vi "2 DOF Helicopter.vi"() -> ()   [LabVIEW 2021]
uses:
  <vilib>/MakerHub/LINX/Public/Sensors/Accelerometer/MPU60X0/DeviceAddresses.ctl
  <vilib>/Simulation/Scripting/Companion Diagram/SimConfigNode/SimParams.ctl
  <vilib>/Simulation/Scripting/Companion Diagram/SimConfigNode/_simSolvers.ctl
  <vilib>/Simulation/Implementation/Shared/SIMSCR Execution Mode.ctl
  <vilib>/Simulation/Param Hierarchy/Typedefs/SIMPH Param Control Actions.ctl
  <vilib>/Simulation/Implementation/Shared/SIM limit type.ctl
  <vilib>/Simulation/Implementation/Shared/NILVSim_ParamChanged.vi
  <vilib>/Simulation/Implementation/Shared/NILVSIM_BeginStep.vi
  <vilib>/Simulation/Utility/Implementation/SIM Halt.vi
  <vilib>/Simulation/SignalArithmetic/Implementation/NILVSim Gain.llb/SIM Gain (scalar).vi
  <vilib>/Simulation/ContinuousLinear/Implementation/NILVSim Derivative.llb/SIM derivative (scalar).vi
  <vilib>/Simulation/SignalDisplay/Implementation/NILVSim Time Waveform.llb/SIM Time Waveform (vector).vi
  <vilib>/Simulation/ContinuousLinear/Implementation/NILVSim Integrator new.llb/SIM Integrator distributor (scalar).vi
  <vilib>/Simulation/ContinuousLinear/Implementation/NILVSim Integrator new.llb/SIM Integrator collector (scalar).vi
  <vilib>/Simulation/Implementation/Shared/SIM Is Init or Final Stage.vi
  <vilib>/MakerHub/LINX/Public/Peripherals/Digital/Digital Write.vi
  <vilib>/MakerHub/LINX/Public/Peripherals/Digital/Digital Write 1 Chan.vi
  <vilib>/MakerHub/LINX/Public/Peripherals/PWM/PWM Set Duty Cycle.vi
  <vilib>/MakerHub/LINX/Public/Peripherals/PWM/PWM Set Duty Cycle 1 Chan.vi
  <vilib>/Simulation/Implementation/Shared/NILVSim_Manager.vi
  <vilib>/Utility/error.llb/Clear Errors.vi
  <vilib>/Simulation/Implementation/Shared/NILVSim_FinalizeModel.vi
  <vilib>/MakerHub/LINX/Public/Peripherals/Digital/Digital Write N Chans.vi
  <vilib>/MakerHub/LINX/Private/Local IO/LinxDigitalWrite.vi
  <vilib>/MakerHub/LINX/Public/Utilities/Check Channel.vi
  <vilib>/MakerHub/LINX/Public/Utilities/Open Serial.vi
  <vilib>/Simulation/Implementation/Shared/SIM Unbundle Sim Info.vi
  <vilib>/Simulation/Implementation/Shared/NILVSim_Initialize.vi
  <vilib>/MakerHub/LINX/Private/Utilties/Generate Error.vi
  <vilib>/MakerHub/LINX/Private/Device/Peripheral/Digital/Digital Write.vi
  <vilib>/MakerHub/LINX/Public/Peripherals/PWM/PWM Set Duty Cycle N Chans.vi
  <vilib>/Simulation/Utility/Implementation/NILVSim Get Time and IsAcceptedStep.vi
  <vilib>/Simulation/Implementation/Shared/SIMSH Read Queue.vi
  <vilib>/Simulation/Implementation/Shared/NILVSim_GetModelError.vi
  <vilib>/Simulation/Implementation/Shared/SIM Bundle Sim Info.vi
  <vilib>/Simulation/Scripting/Companion Diagram/SimConfigNode/SimDog.xnode
  <vilib>/Simulation/Implementation/XNodeFramework/SimXNode/SimX.xnode
  <vilib>/MakerHub/LINX/LMH-LINX.lvlib
  <vilib>/MakerHub/LINX/Public/Sensors/Accelerometer/MPU60X0/MPU60X0.lvlib
  <vilib>/Simulation/ContinuousLinear/Implementation/NILVSim Integrator new.llb/SIM Integrator (scalar).vi
  <vilib>/Simulation/Implementation/Shared/NI_SIM_Implementation.lvlib
panel:
  out "u 2":dbl
  in  "Max 2":dbl=0.9
  in  "Controller 2 ON/OFF":bool
  in  "Gain 2":dbl=15.0
  in  "Kp 2":dbl=24.0
  in  "Ki  2":dbl=1.0
  in  "Kd  2":dbl=0.1
  out "Error Out 2":errorcluster
  out "Waveform Chart":waveform(dbl)[](graph)=[{"t0"=timestamp(2.05 s since 1904-01-01), "dt"=1.0, "Y"=[0.011969439452488623]}, {"t0"=timestamp(2.05 s since 1904-01-01), "dt"=1.0, "Y"=[0.0]}]
  out "Y Axis":i16=574
  in  "Gain":dbl=1.0
  in  "Max":dbl=0.8
  in  "Controller ON/OFF":bool
  out "u":dbl
  out "Iterations":i32=1999
  in  "Iterations":i32=2000
  out "yaw":dbl=0.5188562340966918
  out "Z Axis":i16=1
  out "x/y":dbl=-89.86768864889659
  in  "Halt?":bool
  out "pitch":dbl=0.011969439452488623
  out "Gyro\n Chart 2":T1(graph)={"X Axis"=-479, "Y Axis"=574, "Z Axis"=61}
  out "Acceleration\n Chart":T1(graph)={"X Axis"=4, "Y Axis"=-2344, "Z Axis"=19140}
  out "Acceleration Data (g)":T1={"X Axis"=4, "Y Axis"=-2344, "Z Axis"=19140}
  out "Error Out":errorcluster
  in  "Serial Port":refnum<visa-resource-name>="COM7"
  in  "Kp":dbl=25.0
  in  "Ki":dbl=0.3
  in  "Kd":dbl=0.2
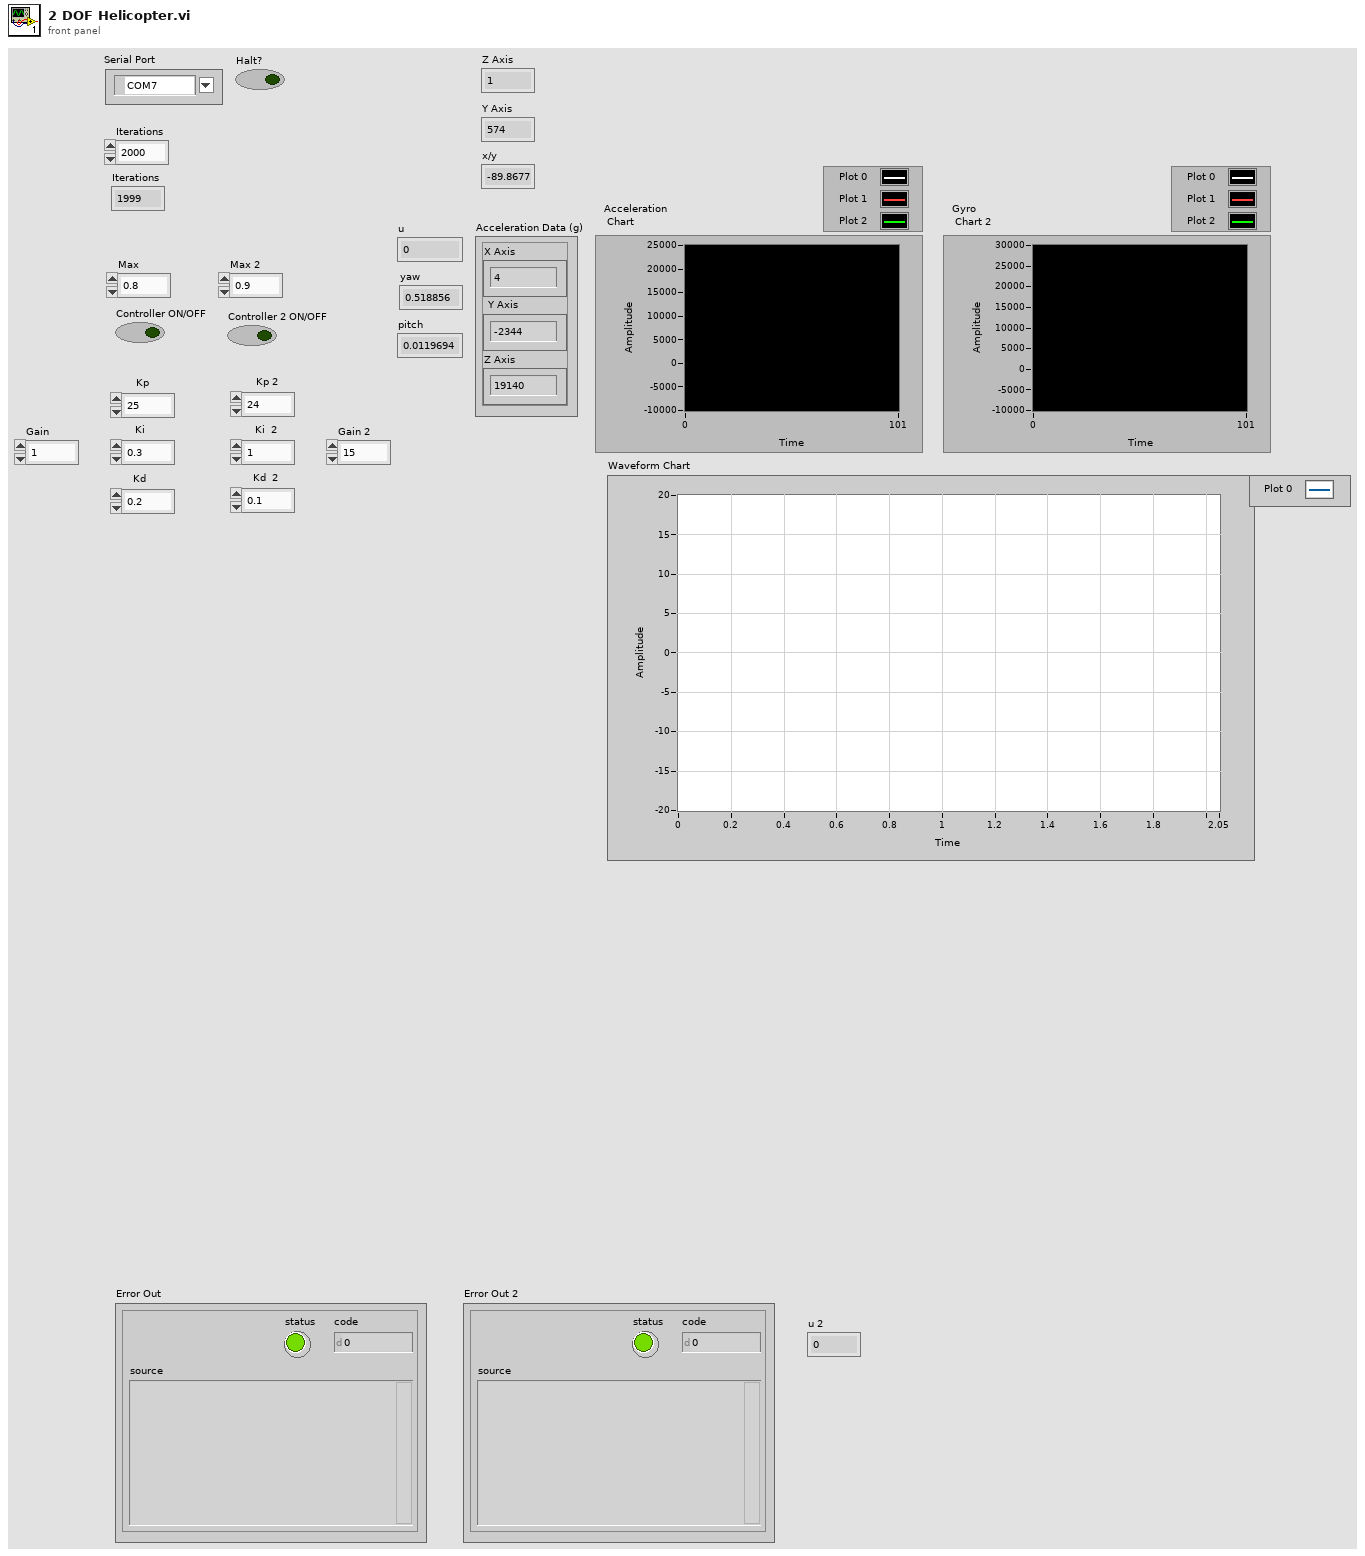
[diagram p1: front panel]
types:
  T1 = cluster{"X Axis":i16, "Y Axis":i16, "Z Axis":i16}
  T2 = typedef "LMH-LINX.lvlib/MPU60X0.lvlib/DeviceAddresses.ctl" = enum16{"0x68", "0x69"}
  T3 = typedef "LMH-LINX.lvlib/LINX Ref.ctl" = cluster{"IO":T4, "Interface":T5, "LINX Device Config":T6}
  T4 = typedef "LMH-LINX.lvlib/Platform.ctl" = enum16{"Remote", "Local"}
  T5 = typedef "LMH-LINX.lvlib/Interface.ctl" = enum16{"Serial", "TCP"}
  T6 = typedef "LMH-LINX.lvlib/Device.lvlib/LINX Device Config.ctl" = cluster{"Interface":T5, "COM Port":refnum<visa-resource-name>, "TCP Configuration":T7, "Device Family":u8, "Device ID":u8, "Device Name":string, "TCP Ref":refnum<k5>, "Channels":T8}
  T7 = typedef "LMH-LINX.lvlib/Device.lvlib/TCP Config.ctl" = cluster{"IP Address":string, "Port":u16}
  T8 = typedef "LMH-LINX.lvlib/Channels.ctl" = cluster{"DI":u8[], "DO":u8[], "AI":u8[], "AO":u8[], "PWM":u8[], "QE":u8[], "UART":u8[], "I2C 2":u8[], "SPI":u8[], "CAN":u8[], "Servo":u8[], "AI Ref (V)":dbl, "AI Resolution (Bits)":u8, "AO Ref (V)":dbl, "AO Resolution (Bits)":u8}
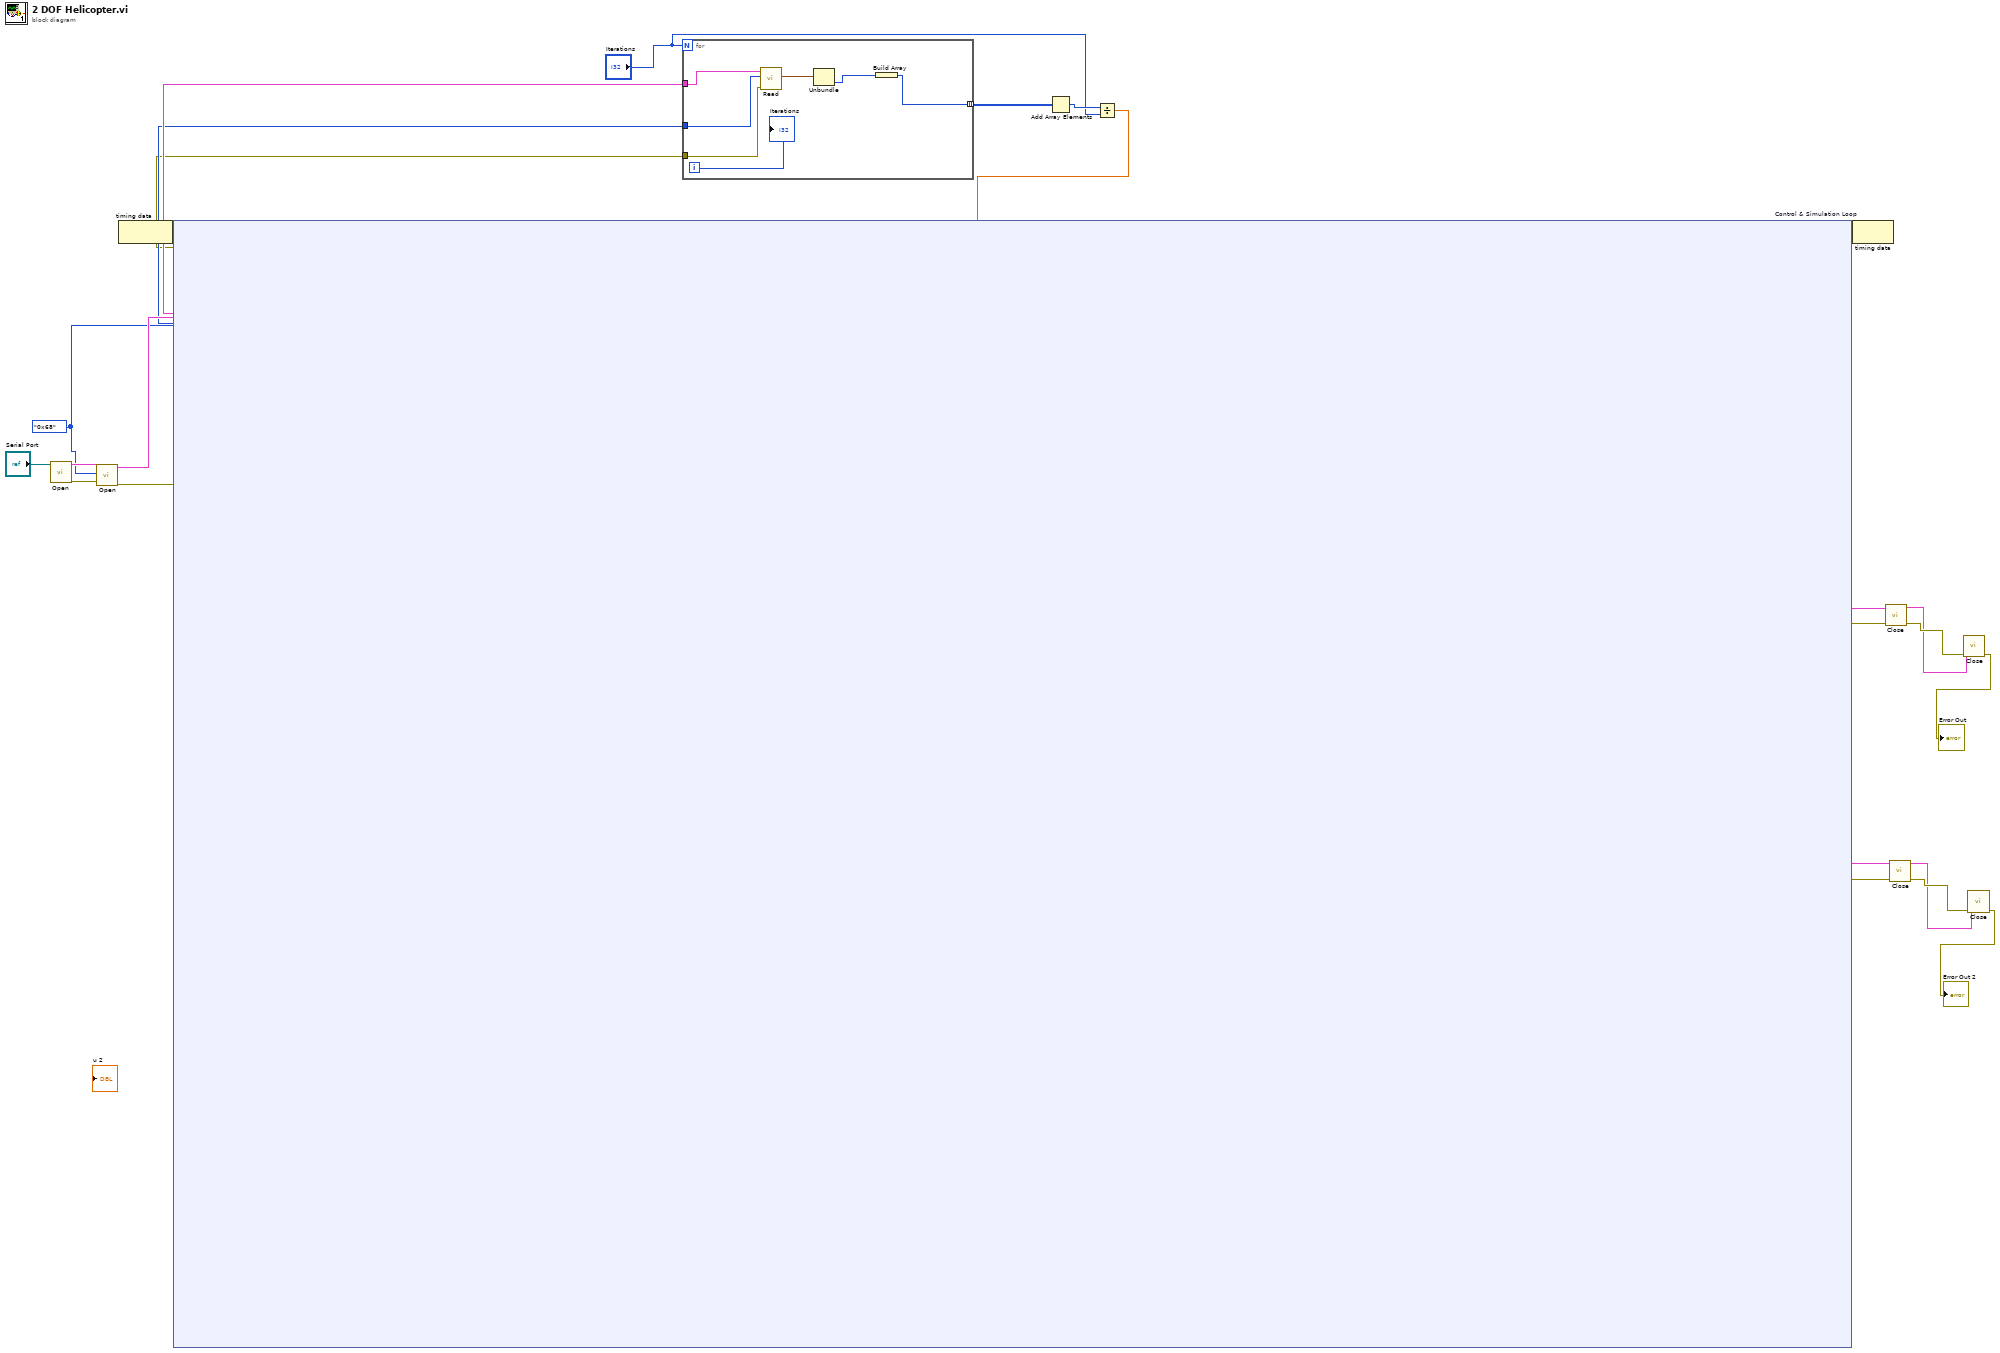
[diagram p0: block diagram]
diagram:
  w11 = DeviceAddresses."0x68" ("I2C Slave Address")
  n1 = call-poly <vilib>:"Open.vi"("Serial Port"="Serial Port") -> ("Error Out"=w20:errorcluster, "LINX Resource"=w21:T3)  [unwired: 8 in, 1 out]
  n2 = call <vilib>:"Open.vi"("Error In"=w20, "I2C Slave Address"=w11, "LINX Resource"=w21) -> ("Error Out"=w10:errorcluster, "LINX Resource"=w12:T3)  [unwired: 7 in]
  n3 = node-c288() -> (w16:variant)  [unwired: 1 in]
  n4 = for {
    N: "Iterations" -> [_]
    tunnel: w12 -> [w28]
    tunnel: w11 -> [w27]
    tunnel: w10 -> [w26]
    tunnel: [w24] -> w9 mode=indexing
    i -> [w29]
    n5 = call <vilib>:"Read.vi"("Error In"=w26, "I2C Slave Address"=w27, "LINX Resource"=w28) -> ("Acceleration Data (g)"=w25:T1)  [unwired: 4 in, 4 out]
    n6 = Unbundle ("Unbundle 2")(w25) -> ("Z Axis"=w23:i16)  [unwired: 2 out]
    n7 = Build Array(w23) -> (w24:i16[])
    "Iterations" <- w29
  }
  n8 = Add Array Elements(numeric array=w9) -> (sum=w8:i16)
  n9 = Divide(x=w8, y="Iterations") -> (x/y=w6:dbl)
  n10 = node-c254 "Control & Simulation Loop"(w16, w12, w10, w11, w6) -> (w15:variant, w14:T3, w13:errorcluster, w2:errorcluster, w1:T3)
  n11 = node-c288(w15) -> ()  [unwired: 1 out]
  n12 = call <vilib>:"Close.vi"("Error In"=w13, "LINX Resource"=w14) -> ("Error Out"=w18:errorcluster, "LINX Resource"=w17:T3)  [unwired: 8 in]
  n13 = call <vilib>:"Close.vi"("Error In"=w2, "LINX Resource"=w1) -> ("Error Out"=w4:errorcluster, "LINX Resource"=w3:T3)  [unwired: 8 in]
  n14 = call <vilib>:"Close.vi"("Error In"=w18, "LINX Resource"=w17) -> ("Error Out"=→"Error Out":errorcluster)  [unwired: 9 in]
  n15 = call <vilib>:"Close.vi"("Error In"=w4, "LINX Resource"=w3) -> ("Error Out"=→"Error Out 2":errorcluster)  [unwired: 9 in]
